vi "Read Multi Eval Meas SEM Extreme Results.vi"(8 "error in (no error)":errorcluster, 10 "Instance (1)":T2=1, 11 "VISA resource name":refnum<visa-resource-name>) -> (0 "error out":errorcluster, 1 "SEM Extreme Results":T1 {"TX Power Max" format="%^.3e"; "TX Power Min" format="%^.3e"; "Occupied Bandwidth" format="%^.3e"}, 2 "Reliability":i32, 3 "VISA resource name out":refnum<visa-resource-name>, 5 "Out Of Tolerance":i32)   [LabVIEW 2020, in "Rohde&Schwarz CMWXP NR FR1 Measurement.lvlib"]
doc: "Return the extreme single value results of the spectrum emission measurement.\n\nAttribute:\nRSCMWXPNRFR1M_ATTR_READ_MULTI_EVAL_MEAS_SEM_EXTREME_RESULTS\n\nRemote-control command:\nREAD:NRSub:MEAS<i>:MEValuation:SEMask:EXTReme?"
uses:
  <instrlib>/Rohde&Schwarz CMWXP NR FR1 Measurement/Rohde&Schwarz CMWXP NR FR1 Measurement.lvlib
  <instrlib>/Rohde&Schwarz CMWXP NR FR1 Measurement/Private/_Instance.ctl
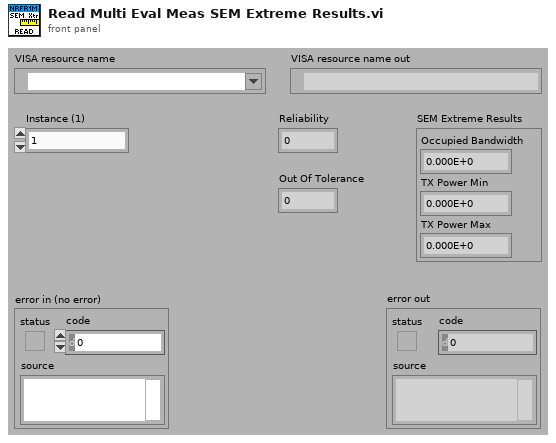
[diagram p1: front panel]
types:
  T1 = cluster{"Occupied Bandwidth":dbl, "TX Power Min":dbl, "TX Power Max":dbl}
  T2 = typedef "Rohde&Schwarz CMWXP NR FR1 Measurement.lvlib/_Instance.ctl" = i32
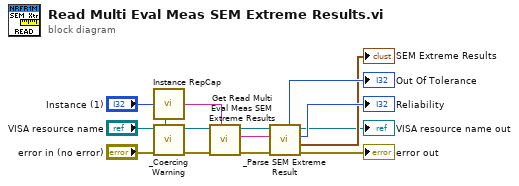
[diagram p0: block diagram]
diagram:
  n1 = call <instrlib>:"Instance RepCap.vi"("Instance In"="Instance (1)") -> ("In Range?"=w12:bool, "RepCap Identifier Out"=w11:string)  [unwired: 1 in]
  n2 = call <instrlib>:"_Coercing Warning.vi"("In Range?"=w12, "error in (no error)"="error in (no error)", "VISA resource name"="VISA resource name") -> ("error out"=w9:errorcluster, "VISA resource name out"=w10:refnum<visa-resource-name>)  [unwired: 7 in]
  n3 = call "Get Read Multi Eval Meas SEM Extreme Results"("Repeated Capabilities"=w11, "error in (no error)"=w9, "instrument handle"=w10) -> ("error out"=w8:errorcluster, "Read Multi Eval Meas SEM Extreme Results"=w6:string, "instrument handle out"=w7:refnum<visa-resource-name>)  [unwired: 6 in]
  n4 = call <instrlib>:"_Parse SEM Extreme Result.vi"("error in (no error)"=w8, "Input String"=w6, "VISA resource name"=w7) -> ("error out"=→"error out":errorcluster, "SEM Extreme Results"=→"SEM Extreme Results":T1, "Reliability"=→"Reliability":i32, "VISA resource name out"=→"VISA resource name out":refnum<visa-resource-name>, "Out Of Tolerance"=→"Out Of Tolerance":i32)  [unwired: 4 in]
